vi "OnDemand_VoltageOutput.vi"(6 "Channel Array":dbl[](array[slide]) scale=0.0..5.067, 9 "minimum voltage":dbl=-5.0 format="%0.2f", 10 "maximum voltage":dbl=5.0 format="%0.2f", 11 "physical channels":tag) -> (0 "error out":errorcluster, 1 "SampClk.Rate":dbl, 2 "number of samples written per channel":u32)   [LabVIEW 2022 SP3]
uses:
  <vilib>/DAQmx/write.llb/DAQmx Write (Analog 1D DBL NChan 1Samp).vi
  <vilib>/DAQmx/create/channels.llb/DAQmx Create Channel (AO-Voltage-Basic).vi
  <vilib>/DAQmx/miscellaneous.llb/DAQmx Fill In Error Info.vi
  <resource>/objmgr/daqmx.rc
panel:
  # "VOLTAGE OUTPUT"
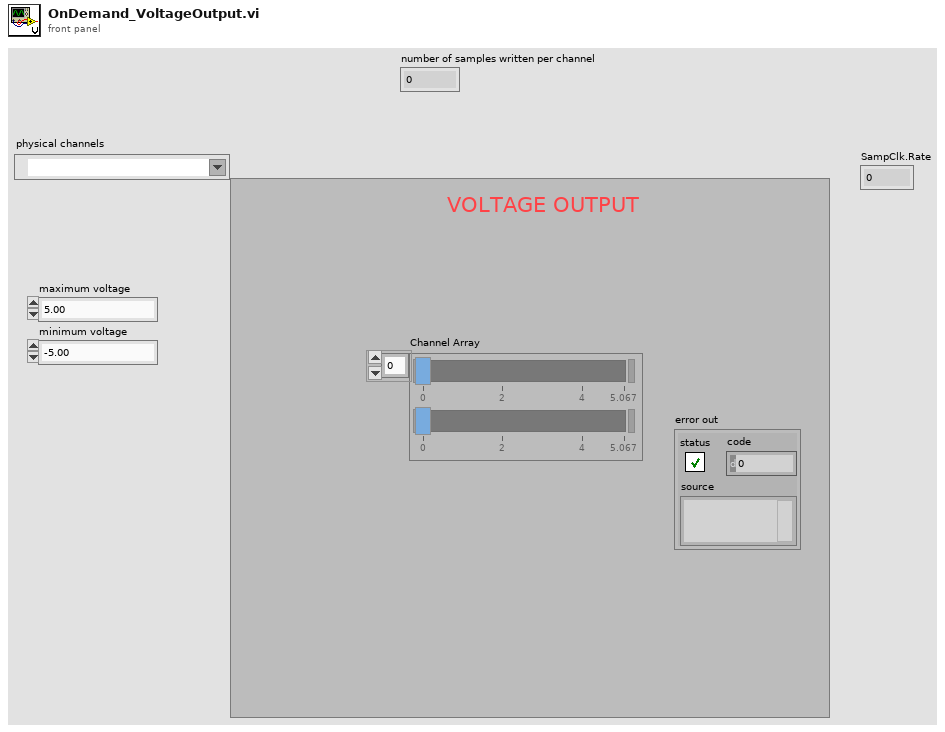
[diagram p1: front panel]
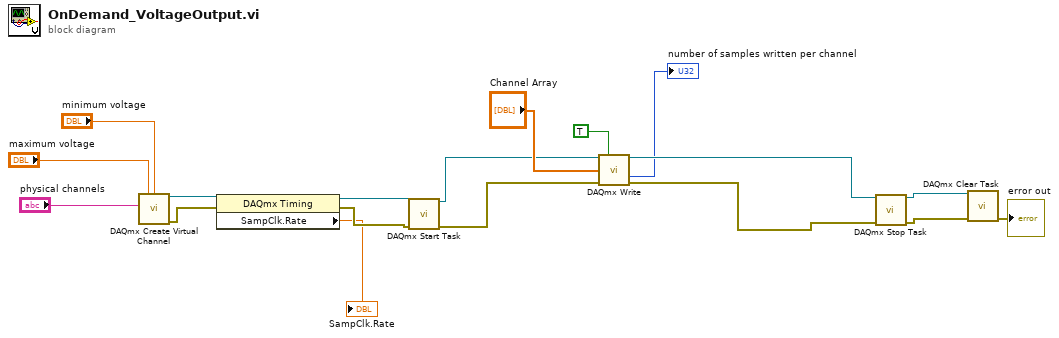
[diagram p0: block diagram]
diagram:
  n1 = call-poly <vilib>:"DAQmx Create Virtual Channel.vi"("maximum value"="maximum voltage", "minimum value"="minimum voltage", "physical channels"="physical channels") -> ("task out"=w4:refnum<k21>, "error out"=w3:errorcluster)  [unwired: 11 in]
  n2 = property class="DAQmx Timing"(reference=w4, error in=w3) -> (reference out=w5:refnum<k21>, error out=w6:errorcluster, "SampClk.Rate"=→"SampClk.Rate":dbl)
  n3 = call <vilib>:"DAQmx Start Task.vi"("task/channels in"=w5, "error in"=w6) -> ("task out"=w12:refnum<k21>, "error out"=w11:errorcluster)  [unwired: 12 in]
  n4 = call-poly <vilib>:"DAQmx Write.vi"("task/channels in"=w12, "auto start"=TRUE, "data"="Channel Array", "error in"=w11) -> ("task out"=w10:refnum<k21>, "number of samples written per channel"=→"number of samples written per channel":u32, "error out"=w9:errorcluster)  [unwired: 9 in]
  n5 = call <vilib>:"DAQmx Stop Task.vi"("task/channels in"=w10, "error in"=w9) -> ("task out"=w16:refnum<k21>, "error out"=w15:errorcluster)  [unwired: 12 in]
  n6 = call <vilib>:"DAQmx Clear Task.vi"("task in"=w16, "error in"=w15) -> ("error out"=→"error out":errorcluster)  [unwired: 13 in]
